vi "U2000_USB_PM_Configure_Units.vi"(7 "Calculate Block (1: Calculate Block 1)":i32(ring)=1 items=["Calculate Block 1"=1, "Calculate Block 2"=2, "Calculate Block 3"=3, "Calculate Block 4"=4], 8 "error in (no error)":errorcluster, 10 "Units (0: dBm)":i32(ring) items=["dBm", "Watts"], 11 "VISA resource name":refnum<visa-resource-name>) -> (0 "error out":errorcluster, 3 "VISA resource name out":refnum<visa-resource-name>)   [LabVIEW 2015]
doc: "Specifies the unit to which the power value is converted after measurement."
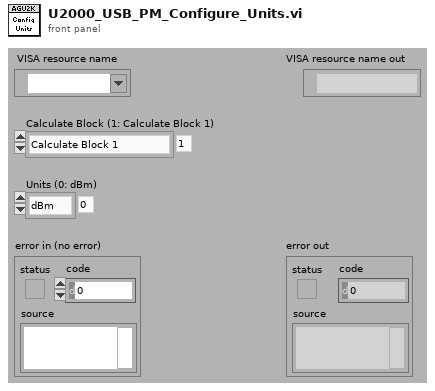
[diagram p1: front panel]
types:
  T1 = typedef "U20xx_USB_PM_User_Data_Out.ctl" = cluster{"U2000 Series Mode":u16, "Trigger Source Int/Ext":bool}
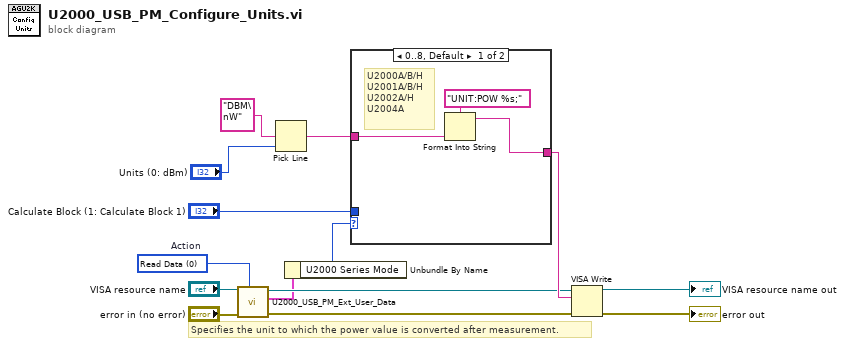
[diagram p0: block diagram]
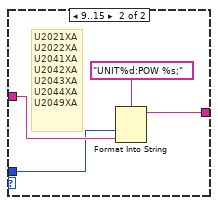
[diagram p2: hidden frame]
diagram:
  w3 = 0 items=["Read Data", "Write Data", "Clear Data", "Clear ALL Data"]  # Action
  # "Specifies the unit to which the power value is converted after measurement."
  n1 = call "U2000_USB_PM_Ext_User_Data.vi"("Action (1: Write Data)"=w3, "error in (no error)"="error in (no error)", "VISA resource name"="VISA resource name") -> ("error out"=w4:errorcluster, "User Data Out"=w2:T1, "VISA resource name out"=w5:refnum<visa-resource-name>)  [unwired: 6 in]
  n2 = Pick Line(multi-line string="DBM\nW", line index="Units (0: dBm)") -> (output string=w9:string)  [unwired: 1 out]
  n3 = Unbundle By Name(w2) -> ("U2000 Series Mode"=w1:u16)
  n4 = case shown="0..8, Default" w1 {
    tunnel: "Calculate Block (1: Calculate Block 1)" -> [_ w19]
    tunnel: w9 -> [w15 w20]
    tunnel: [w16 w18] -> w8
    frame 0..8, Default {
      # "U2000A/B/H\nU2001A/B/H\nU2002A/H\nU2004A"
      n5 = Format Into String(format string="UNIT:POW %s;", w15) -> (resulting string=w16:string)  [unwired: 2 in, 1 out]
    }
    frame 9..15 {
      # "U2021XA\nU2022XA\nU2041XA\nU2042XA\nU2043XA\nU2044XA\nU2049XA"
      n6 = Format Into String(format string="UNIT%d:POW %s;", w19, w20) -> (resulting string=w18:string)  [unwired: 2 in, 1 out]
    }
  }
  n7 = VISA Write(VISA resource name=w5, write buffer=w8, error in (no error)=w4) -> (VISA resource name out=→"VISA resource name out":refnum<visa-resource-name>, error out=→"error out":errorcluster)  [unwired: 1 out]
